vi "Decimal_a_GMS.vi"(0 "Decimal":dbl) -> (1 "Grados":i32, 2 "Minutos":i32, 3 "Segundos":i32)   [LabVIEW 2020]
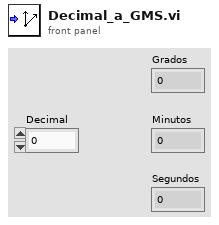
[diagram p1: front panel]
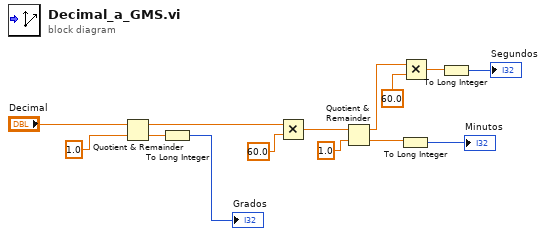
[diagram p0: block diagram]
diagram:
  n1 = Quotient & Remainder(x="Decimal", y=1.0) -> (x-y*floor(x/y)=w10:dbl, floor(x/y)=w12:dbl)
  n2 = To Long Integer(number=w12) -> (32bit integer=→"Grados":i32)
  n3 = Multiply(x=w10, y=60.0) -> (x*y=w8:dbl)
  n4 = Quotient & Remainder(x=w8, y=1.0) -> (x-y*floor(x/y)=w4:dbl, floor(x/y)=w6:dbl)
  n5 = To Long Integer(number=w6) -> (32bit integer=→"Minutos":i32)
  n6 = Multiply(x=w4, y=60.0) -> (x*y=w2:dbl)
  n7 = To Long Integer(number=w2) -> (32bit integer=→"Segundos":i32)
